vi "Read Description.vi"(11 "House Blend in":refnum<class "House Blend.lvclass">) -> (2 "Description":string)   [LabVIEW 2013, in "House Blend.lvclass"]
uses:
  House Blend.lvclass
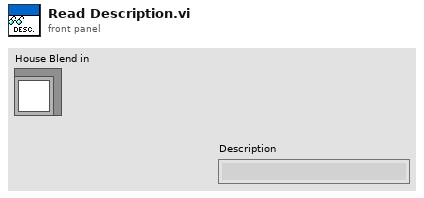
[diagram p1: front panel]
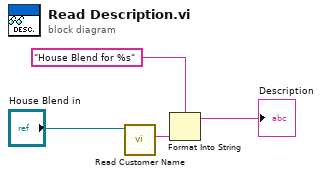
[diagram p0: block diagram]
diagram:
  n1 = call-dynamic "Read Customer Name.vi"("Beverage in"="House Blend in") -> ("Customer Name"=w4:string)  [unwired: 10 in]
  n2 = Format Into String(format string="House Blend for %s", w4) -> (resulting string=→"Description":string)  [unwired: 2 in, 1 out]
